vi "Search Sub-Sections.vi"(8 "error in":errorcluster, 9 "Count":u8, 10 "Parent Section":refnum<class "Section Name.lvclass">, 11 "Dictionary in":refnum<class "Dictionary.lvclass">) -> (0 "error out":errorcluster, 1 "Found":u8, 2 "Sub-Sections":refnum<class "Section.lvclass">[](array[class]), 3 "Dictionary out":refnum<class "Dictionary.lvclass">)   [LabVIEW 2024, in "Electronic Datasheet.lvlib" / "Dictionary.lvclass"]
uses:
  Dictionary.lvclass
  Section Name/Section Name.lvclass
  OD Section/Section.lvclass
  Dictionary.lvclass/Dictionary.ctl
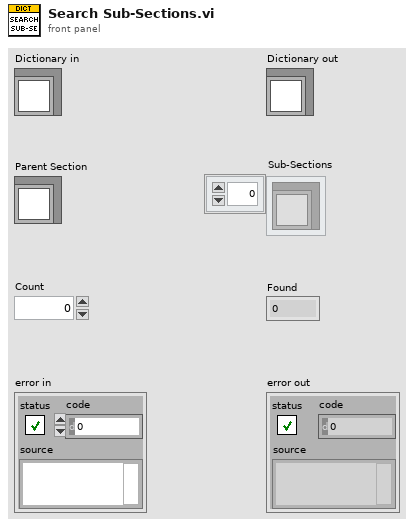
[diagram p1: front panel]
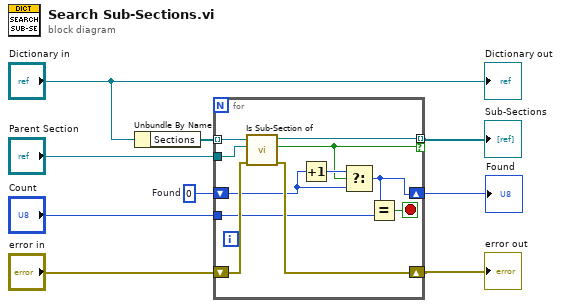
[diagram p0: block diagram]
diagram:
  w4 = u8 0  # Found
  n1 = Unbundle By Name("Dictionary in") -> ("Sections"=w9:refnum<class "Section.lvclass">[])
  n2 = for {
    tunnel: w9 -> [w18] mode=indexing
    tunnel: [w20] -> w1 mode=indexing if=w10
    tunnel: "Parent Section" -> [w19]
    shift-right: [w16] -> w5
    shift-left: "error in" -> [w17]
    shift-right: [w11] -> w2
    shift-left: w4 -> [w14]
    tunnel: "Count" -> [w12]
    stop <- w13 stop-if-true
    n3 = call "Is Sub-Section of.vi"("error in"=w17, "Parent Section Name"=w19, "Section in"=w18) -> ("error out"=w16:errorcluster, "Is Sub-Section?"=w10:bool, "Section out"=w20:refnum<class "Section.lvclass">)  [unwired: 6 in]
    n4 = Increment(x=w14) -> (x+1=w15:u8)
    n5 = Select(t=w15, s=w10, f=w14) -> (s? t:f=w11:u8)
    n6 = Equal?(x=w11, y=w12) -> (x = y?=w13:bool)
  }
  "error out" <- w5
  "Found" <- w2
  "Sub-Sections" <- w1
  "Dictionary out" <- "Dictionary in"
